vi "Remove NaN for Fit.vi"(3 "Data in":dbl[](array[numeric])) -> (0 "Weight out":dbl[](array[numeric]), 1 "Data out":dbl[](array[numeric]))   [LabVIEW 2016, in "Abstract Fit.lvclass"]
uses:
  Abstract Fit.lvclass
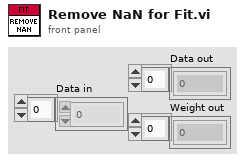
[diagram p1: front panel]
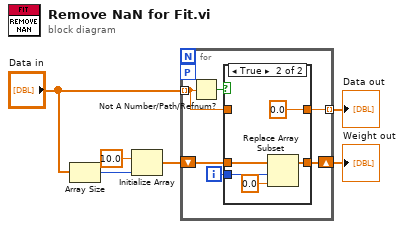
[diagram p0: block diagram]
diagram:
  n1 = Array Size(array="Data in") -> (size(s)=w5:i32)
  n2 = Initialize Array(10.0 ("element"), w5) -> (w3:dbl[])
  n3 = for {
    tunnel: "Data in" -> [w8] mode=indexing
    shift-right: [w10] -> w1
    shift-left: w3 -> [w11]
    tunnel: [w7] -> w2 mode=indexing
    workers-P: _ -> [_]
    i -> [w9]
    n4 = Not A Number/Path/Refnum?(number/path/refnum=w8) -> (NaN/Path/Refnum?=w12:bool)
    n5 = case shown="True" w12 {
      tunnel: w11 -> [w13 w19]
      tunnel: [w13 w15] -> w10
      tunnel: w9 -> [_ w17]
      tunnel: w8 -> [w14 _]
      tunnel: [w14 0.0] -> w7
      frame False {
      }
      frame True {
        n6 = Replace Array Subset(array=w19, new element=0.0 ("new element/subarray"), index=w17) -> (w15:dbl[])
      }
    }
  }
  "Data out" <- w2
  "Weight out" <- w1
